vi "COM.vi"(3 "Read?":bool=TRUE, 4 "Write?":bool, 5 "command":string, 6 "VISA in":refnum<visa-resource-name>="COM1") -> (0 "nbytes":u32=2, 1 "reply":string="> ", 2 "VISA out":refnum<visa-resource-name>="COM1")   [LabVIEW 2022 SP3]
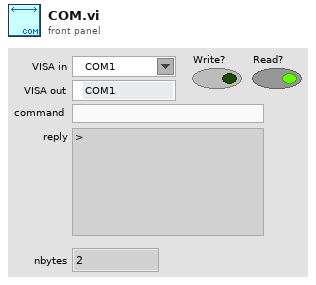
[diagram p1: front panel]
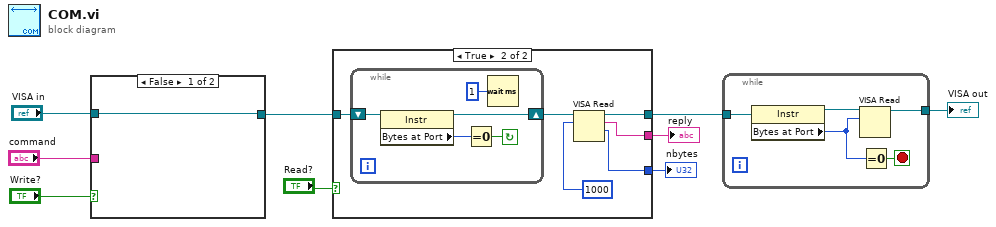
[diagram p0: block diagram]
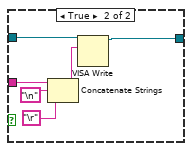
[diagram p2: hidden frame]
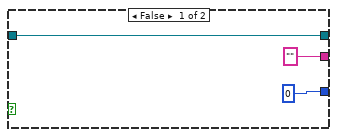
[diagram p3: hidden frame]
diagram:
  n1 = case shown="False" "Write?" {
    tunnel: "command" -> [_ w14]
    tunnel: "VISA in" -> [w10 w16]
    tunnel: [w10 w15] -> w7
    frame False {
    }
    frame True {
      n2 = Concatenate Strings(w14, "\n", "\r") -> (w13:string)
      n3 = VISA Write(VISA resource name=w16, write buffer=w13) -> (VISA resource name out=w15:refnum<visa-resource-name>)  [unwired: 1 in, 2 out]
    }
  }
  n4 = case shown="True" "Read?" {
    tunnel: ["" ("read buffer") w25] -> w8
    tunnel: w7 -> [w18 w24]
    tunnel: [w18 w22] -> w2
    tunnel: [u32 0 ("return count") w21] -> w3
    frame False {
    }
    frame True {
      n5 = while {
        shift-right: [w29] -> w23
        shift-left: w24 -> [w30]
        stop <- w28 continue-if-true
        n6 = property class="Instr"(reference=w30) -> (reference out=w29:refnum<visa-resource-name>, "Bytes at Port"=w27:u32)  [unwired: 1 in, 1 out]
        n7 = Equal To 0?(x=w27) -> (x = 0?=w28:bool)
        n8 = Wait (ms)(milliseconds to wait=u32 1) -> ()  [unwired: 1 out]
      }
      n9 = VISA Read(VISA resource name=w23, byte count=u32 1000) -> (VISA resource name out=w22:refnum<visa-resource-name>, read buffer=w25:string, return count=w21:u32)  [unwired: 1 in, 1 out]
    }
  }
  "reply" <- w8
  "nbytes" <- w3
  n10 = while {
    tunnel: w2 -> [w35]
    tunnel: [w31] -> w1
    stop <- w32 stop-if-true
    n11 = property class="Instr"(reference=w35) -> (reference out=w34:refnum<visa-resource-name>, "Bytes at Port"=w33:u32)  [unwired: 1 in, 1 out]
    n12 = VISA Read(VISA resource name=w34, byte count=w33) -> (VISA resource name out=w31:refnum<visa-resource-name>)  [unwired: 1 in, 3 out]
    n13 = Equal To 0?(x=w33) -> (x = 0?=w32:bool)
  }
  "VISA out" <- w1
